vi "Adaptive Noise Cancellation (Host).vi"() -> ()   [LabVIEW 2023]
doc: "This VI is the host VI of the adaptive noise cancellation. Run this VI on the host PC. Refer to the description of the Adaptive Noise Cancellation.proj file for more information. The Adaptive Noise Cancellation project contains this VI."
uses:
  <vilib>/rvi/interface/nirviMethod/nirviMethod.xnode
  <vilib>/rvi/interface/nirviReadWriteControl/nirviReadWriteControl.xnode
  <vilib>/Platform/TimedLoop/XDataNode/XDataNode.xnode
  <vilib>/Platform/TimedLoop/XDataNode/nitl_modes.ctl
  <vilib>/Platform/TimedLoop/XDataNode/XDNodeRunTimeDep.lvlib
  <vilib>/Platform/TimedLoop/XDataNode/wakeup.ctl
  <vilib>/Platform/TimedLoop/XDataNode/timing_clust.ctl
  <vilib>/rvi/interface/nirviOpenFPGA/nirviOpenFPGA.xnode
  <vilib>/sound/lvsound.llb/Sound Format.ctl
  <vilib>/Analysis/NI_AALPro.lvlib
  <vilib>/Analysis/2dsp.llb/Rational Resample (single channel, DBL).vi
  <vilib>/rvi/interface/nirviCloseFPGA/nirviCloseFPGA.xnode
  FPGA Bitfiles/adaptivenoisecan_FPGATarget_AdaptiveNoiseCan_JEhy1BWumyw.lvbitx
  Adaptive Noise Cancellation (FPGA).vi
  <vilib>/rvi/errors/niLvFpgaMergeErrorWithErrorCode.vi
  <vilib>/userdefined/High Color/nirio_resource_hc.ctl
panel:
  in  "Tab Control":T1(tab)
  in  "Sound to Play":enum16{"Before ANC", "After ANC"}(ring)
  out "Before Adaptive Noise Cancellation":waveform(dbl)(graph)
  in  "Volume":dbl(slide)=20.0 scale=0.0..100.0
  in  "Stop":bool
  in  "Reset":bool
  out "After Adaptive Noise Cancellation":waveform(dbl)(graph)
  in  "RIO Device":T2
  in  "Step Size":fxp<+/-,16,-1>=0.01000213623046875 format="%.5g"
  # "Refer to the Adaptive Noise Cancellation topic in the LabVIEW Help for more information about the background of adaptive noise cancellation. Select Help>>Show Context Help and move the cursor over the VI icon for more information about this example."
  # "Connection Diagram"
  # "Theoretical Diagram"
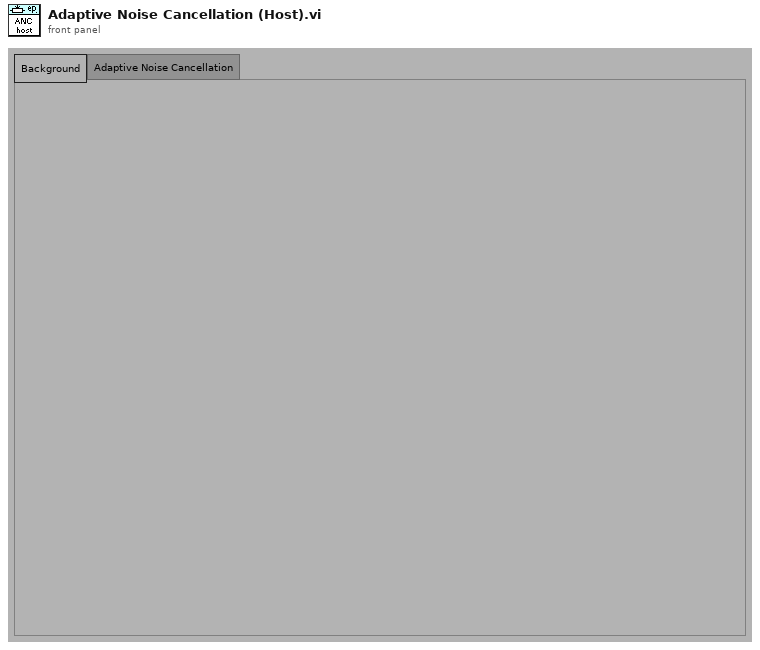
[diagram p1: front panel]
types:
  T1 = enum32{"Background", "Adaptive Noise Cancellation"}
  T2 = typedef "nirio_resource_hc.ctl" = tag
  T3 = typedef "Sound Format.ctl" = cluster{"sound quality":enum16{"mono", "stereo"}, "rate":enum16{"11025", "22050", "44100", "8000"}, "bits per sample":enum16{"8 bit", "16 bit"}}
  T4 = typedef "XDNodeRunTimeDep.lvlib/timing_clust.ctl" = cluster{"Expected End [f-1]":u64, "Actual End [f-1]":u64, "Finished Late? [f-1]":bool, "Expected End [i-1]":u64, "Actual End [i-1]":u64, "Finished Late? [i-1]":bool, "Expected Start [i]":u64, "Actual Start [i]":u64, "Expected Start [f]":u64, "Actual Start [f]":u64, "Source Name":string, "Structure Name":string, "Period":i64, "Deadline":i64, "Offset":i64, "Start":i64, "Priority":i32, "Timeout":i32, "Mode":T5, "Wakeup Reason":T6, "Error":errorcluster, "Source Type":string, "Secondary Source Type":string, "Global End Time":u64, "Global Start Time":u64, "Frame Duration":u64, "Iteration Duration":u64, "Assigned CPU":i32, "I/O Scan Engine Mode":u32}
  T5 = typedef "XDNodeRunTimeDep.lvlib/nitl_modes.ctl" = enum32{"No Change", "Process missed periods, maintain original phase", "Discard missed periods, maintain original phase", "Process missed periods, ignore original phase", "Discard missed periods, ignore original phase"}
  T6 = typedef "XDNodeRunTimeDep.lvlib/wakeup.ctl" = enum32{"Normal", "Aborted", "Asynchronous wakeup", "Timing source error", "Timed loop error", "Timeout"}
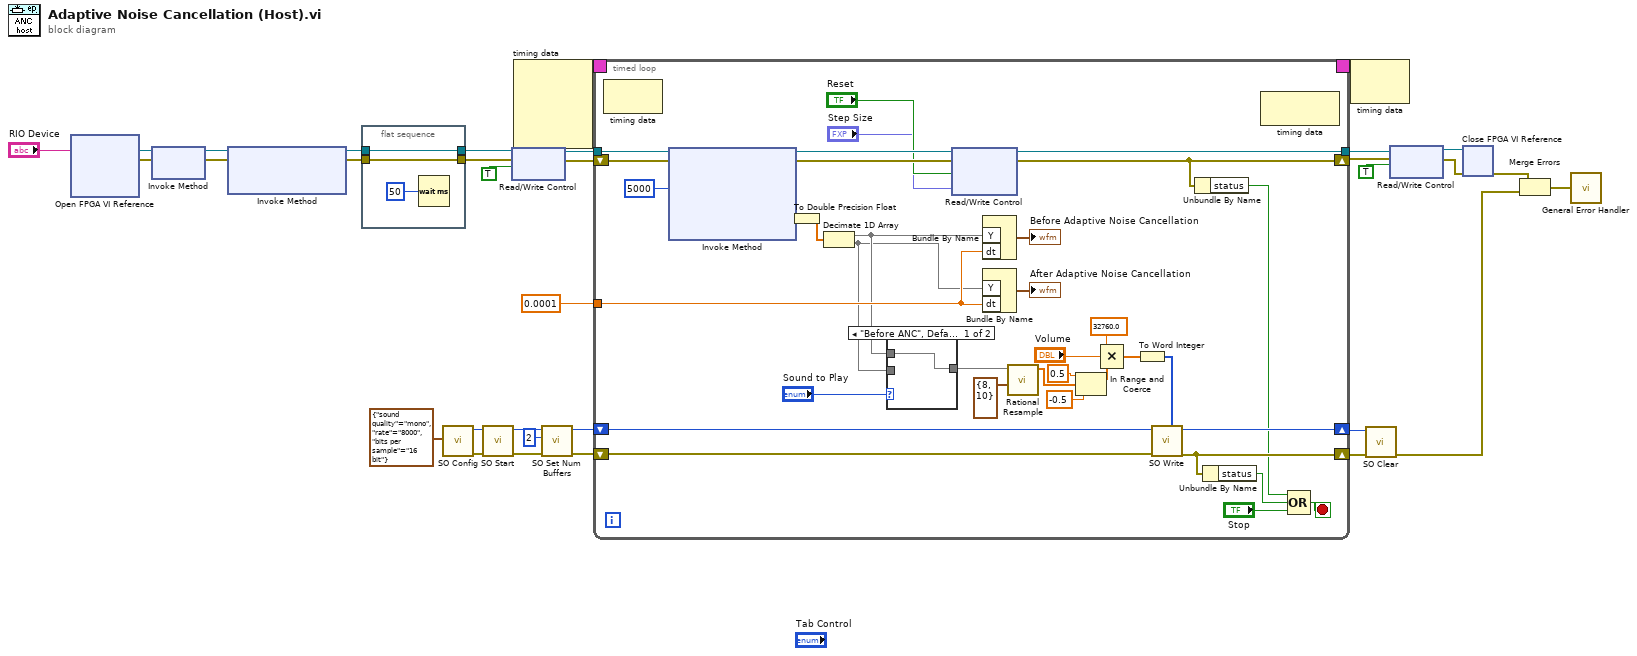
[diagram p0: block diagram]
diagram:
  n1 = xnode "Open FPGA VI Reference"("resource name"="RIO Device") -> ("FPGA VI Reference Out"=w29:refnum<k20>, "error out"=w28:errorcluster)  [unwired: 1 in]
  n2 = xnode "Invoke Method"("FPGA VI Reference In"=w29, "error in"=w28) -> ("FPGA VI Reference Out"=w26:refnum<k20>, "error out"=w25:errorcluster)
  n3 = xnode "Invoke Method"("FPGA VI Reference In"=w26, "error in"=w25) -> ("FPGA VI Reference Out"=w5:refnum<k20>, "error out"=w4:errorcluster)  [unwired: 1 in]
  n4 = flat-sequence {
    tunnel: w5 -> [w35]
    tunnel: [w35] -> w8
    tunnel: w4 -> [w34]
    tunnel: [w34] -> w7
    frame #0 {
      n5 = Wait (ms)(milliseconds to wait=u32 50) -> ()  [unwired: 1 out]
    }
  }
  n6 = call <vilib>:"SO Config.vi"("sound format"=T3 {"sound quality"=enum."mono", "rate"=enum."8000", "bits per sample"=enum."16 bit"}) -> ("error out"=w21:errorcluster, "task ID out"=w20:u32)  [unwired: 1 in, 8 out]
  n7 = call <vilib>:"SO Start.vi"("error in (no error)"=w21, "task ID in"=w20) -> ("error out"=w24:errorcluster, "task ID out"=w23:u32)  [unwired: 8 out]
  n8 = xnode "Read/Write Control"("FPGA VI Reference In"=w8, "error in"=w7, "start"=TRUE) -> ("FPGA VI Reference Out"=w30:refnum<k20>, "error out"=w27:errorcluster)
  n9 = node-c288() -> (w33:T4)  [unwired: 4 out]
  n10 = call <vilib>:"SO Set Num Buffers.vi"("error in (no error)"=w24, "number of buffers"=2, "task ID in"=w23) -> ("error out"=w17:errorcluster, "task ID out"=w18:u32)  [unwired: 7 out]
  n11 = timed-loop {
    timing: w33 -> [_]
    timing-out: [_] -> w32
    tunnel: w30 -> [w71]
    tunnel: [w67] -> w13
    shift-right: [w41] -> w12
    shift-left: w27 -> [w69]
    tunnel: 0.0001 -> [w59]
    shift-right: [w64] -> w16
    shift-left: w18 -> [w61]
    shift-right: [w40] -> w15
    shift-left: w17 -> [w60]
    stop <- w39 stop-if-true
    n12 = node-c288() -> ()  [unwired: 2 out]
    n13 = xnode "Invoke Method"("FPGA VI Reference In"=w71, "error in"=w69, "Number of Elements"=u32 5000) -> ("FPGA VI Reference Out"=w68:refnum<k20>, "error out"=w66:errorcluster, "Data"=w49:void[])  [unwired: 1 in, 1 out]
    n14 = To Double Precision Float(number=w49) -> (double precision float=w48:dbl[])
    n15 = Decimate 1D Array(w48) -> (w43:dbl[], w42:dbl[])
    n16 = case shown="\"Before ANC\", Default" "Sound to Play" {
      tunnel: [w72 w73] -> w44
      tunnel: w43 -> [w72 _]
      tunnel: w42 -> [_ w73]
      frame "Before ANC", Default {
      }
      frame "After ANC" {
      }
    }
    n17 = xnode "Read/Write Control"("FPGA VI Reference In"=w68, "error in"=w66, "reset? (F)"="Reset", "step size"="Step Size") -> ("FPGA VI Reference Out"=w67:refnum<k20>, "error out"=w41:errorcluster)
    n18 = Bundle By Name("Y"=w43, "dt"=w59) -> (→"Before Adaptive Noise Cancellation":waveform(dbl))  [unwired: 1 out]
    n19 = Bundle By Name("Y"=w42, "dt"=w59) -> (→"After Adaptive Noise Cancellation":waveform(dbl))  [unwired: 1 out]
    n20 = call-poly <vilib>:"Rational Resample.vi"("resample factor"=cluster{"interpolation":i32, "decimation":i32} {"interpolation"=8, "decimation"=10}, "X"=w44) -> ("Y"=w53:dbl[])  [unwired: 5 in, 4 out]
    n21 = In Range and Coerce(upper limit=0.5, x=w53, lower limit=-0.5) -> (coerced(x)=w52:dbl[])  [unwired: 1 out]
    n22 = Compound Arithmetic op=MULTIPLY(32760.0 ("Volume 2"), "Volume", w52) -> (w62:dbl[])
    n23 = To Word Integer(number=w62) -> (16bit integer=w46:i16[])
    n24 = call <vilib>:"SO Write.vi"("mono 16-bit"=w46, "error in (no error)"=w60, "task ID in"=w61) -> ("error out"=w40:errorcluster, "task ID out"=w64:u32)  [unwired: 3 in, 4 out]
    n25 = Unbundle By Name(w41) -> ("status"=w37:bool)
    n26 = Unbundle By Name(w40) -> ("status"=w38:bool)
    n27 = node-c288() -> ()  [unwired: 2 out]
    n28 = Compound Arithmetic op=OR(w37, w38, "Stop") -> (w39:bool)
  }
  n29 = node-c288(w32) -> ()  [unwired: 1 out]
  n30 = call <vilib>:"SO Clear.vi"("error in (no error)"=w15, "task ID in"=w16) -> ("error out"=w2:errorcluster)  [unwired: 9 out]
  n31 = xnode "Read/Write Control"("FPGA VI Reference In"=w13, "error in"=w12, "stop"=TRUE) -> ("FPGA VI Reference Out"=w10:refnum<k20>, "error out"=w9:errorcluster)
  n32 = xnode "Close FPGA VI Reference"("FPGA VI Reference In"=w10, "error in"=w9) -> ("error out"=w3:errorcluster)
  n33 = Merge Errors(w3, w2) -> (w1:errorcluster)
  n34 = call <vilib>:"General Error Handler.vi"("error in (no error)"=w1) -> ()  [unwired: 2 in, 13 out]
